vi "Get Port.vi"(8 "error in (no error)":errorcluster, 11 "URI in":refnum<class "URI.lvclass">) -> (0 "error out":errorcluster, 2 "Port":u16, 3 "URI out":refnum<class "URI.lvclass">)   [LabVIEW 2020, in "URI.lvclass"]
uses:
  URI.lvclass
  URI.lvclass/URI.ctl
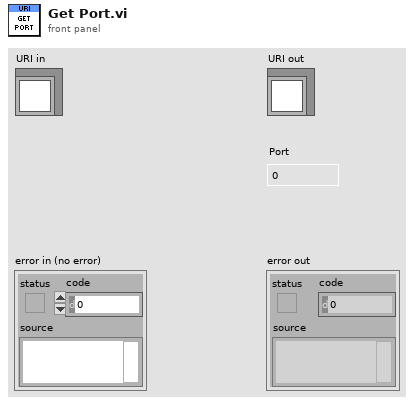
[diagram p1: front panel]
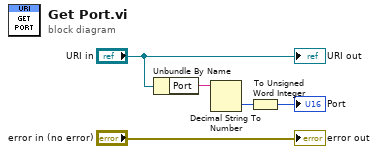
[diagram p0: block diagram]
diagram:
  n1 = Unbundle By Name("URI in") -> ("Port"=w3:string)
  n2 = Decimal String To Number(string=w3) -> (number=w2:i32)  [unwired: 2 in, 1 out]
  n3 = To Unsigned Word Integer(number=w2) -> (unsigned 16bit integer=→"Port":u16)
  "error out" <- "error in (no error)"
  "URI out" <- "URI in"
